vi "Global_Library Path.vi"() -> ()   [LabVIEW 2020, in "AIM ARINC 429 Hardware API.lvlib"]
uses:
  AIM ARINC 429 Hardware API.lvlib
panel:
  in  "library path":path
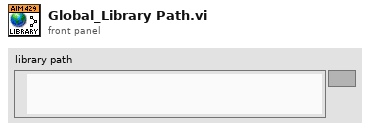
[diagram p1: front panel]
diagram:
